vi "Batch table.vi"() -> (3 "Batch table":string)   [LabVIEW 2024]
uses:
  CTRLS/GLB_VAR.vi
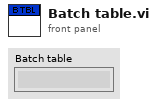
[diagram p1: front panel]
types:
  T1 = typedef "REF.ctl" = cluster{"Save Settings":refnum<vi>, "Navigation":refnum<vi>, "Main Tab":refnum<vi>, "Password":refnum<vi>, "BatchData":refnum<vi>, "Serial Data":refnum<vi>, "Username":refnum<vi>, "Stop Printing":refnum<vi>, "Run statistics":refnum<vi>, "System settings":refnum<vi>, "Batch Managment contol":refnum<vi>, "Start Printing":refnum<vi>, "BatchData MNG":refnum<vi>, "MSG Cenetr":refnum<vi>, "Printer status":refnum<vi>, "Printer Message Config":refnum<vi>, "Ready and Paused Batches":refnum<vi>, "Camera Setup":refnum<vi>, "Batch statistics":refnum<vi>, "Logout":refnum<vi>}
  T2 = typedef "Open Batch Data.ctl" = cluster{"Batch Name":string, "Batch Number":string, "GTIN":string, "Expiry Date":string, "MFG Date":string}
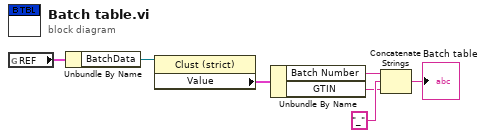
[diagram p0: block diagram]
diagram:
  n1 = global read "GLB_VAR.vi" "REF"() -> (w1:T1)
  n2 = Unbundle By Name(w1) -> ("BatchData"=w3:refnum<vi>)
  n3 = property class="Clust (strict)"(reference=w3) -> ("Value"=w4:T2)  [unwired: 1 in, 2 out]
  n4 = Unbundle By Name(w4) -> ("Batch Number"=w5:string, "GTIN"=w6:string)
  n5 = Concatenate Strings(w5, "_" ("string"), w6) -> (→"Batch table":string)
